vi "get_errorCluster.vi"(1 "HGF_Exception":refnum<class "HGF_Exception.lvclass">) -> (0 "errorCluster":errorcluster, 2 "dup HGF_Exception":refnum<class "HGF_Exception.lvclass">)   [LabVIEW 2014, in "HGF_BaseClasses.lvlib" / "HGF_Exception.lvclass"]
doc: "This VI retruns the errorCluster attribute."
uses:
  HGF_Exception.lvclass
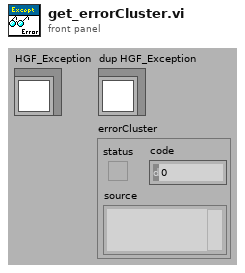
[diagram p1: front panel]
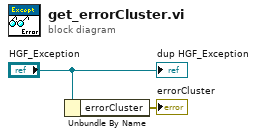
[diagram p0: block diagram]
diagram:
  n1 = Unbundle By Name("HGF_Exception") -> ("errorCluster"=→"errorCluster":errorcluster)
  "dup HGF_Exception" <- "HGF_Exception"
